vi "main_mg400_m1pro.vi"() -> ()   [LabVIEW 2017]
panel:
  out "error out 6":errorcluster
  in  "MoveL":bool
  out "error out 5":errorcluster
  out "error out 4":errorcluster
  out "error out 3":errorcluster
  out "Current SpeedFactor":dbl
  out "error out 2":errorcluster
  out "Error Log":string
  in  "GetErrorID":bool
  out "x value":string
  out "y value":string
  out "z value":string
  out "rx value":string
  out "j4 value":string
  out "j3 value":string
  out "j2 value":string
  out "j1 value":string
  in  "rx-":bool
  in  "z-":bool
  in  "y-":bool
  in  "x-":bool
  in  "rx+":bool
  in  "z+":bool
  in  "y+":bool
  in  "x+":bool
  in  "JointMovJ":bool
  in  "j4":dbl
  in  "j3":dbl
  in  "j2":dbl
  in  "j1":dbl
  in  "Reset Robot":bool
  in  "Feedback Port":string="30004"
  in  "Move Port":string="30003"
  in  "Dashboard Port":string="29999"
  in  "IP Address":string="192.168.5.1"
  in  "stop get state":bool
  out "state error out 2":errorcluster
  out "Robot mode":T1(ring)
  out "speed set string":string
  in  "j4-":bool
  in  "j3-":bool
  in  "j2-":bool
  in  "j1-":bool
  in  "j4+":bool
  in  "j3+":bool
  in  "j2+":bool
  in  "j1+":bool
  out "error out":errorcluster
  in  "stop connect":bool
  in  "Start trace":bool
  in  "tracePath":string
  in  "Stop move":bool
  in  "MoveJ":bool
  in  "rx":dbl
  in  "z":dbl
  in  "y":dbl
  in  "x":dbl
  in  "Speed confrim":bool
  in  "Speed Ratio":dbl=50.0
  in  "Emergency Stop":bool
  in  "Power up":bool
  out "Log":string
  in  "ClearError":bool
  in  "Enable Robot":bool
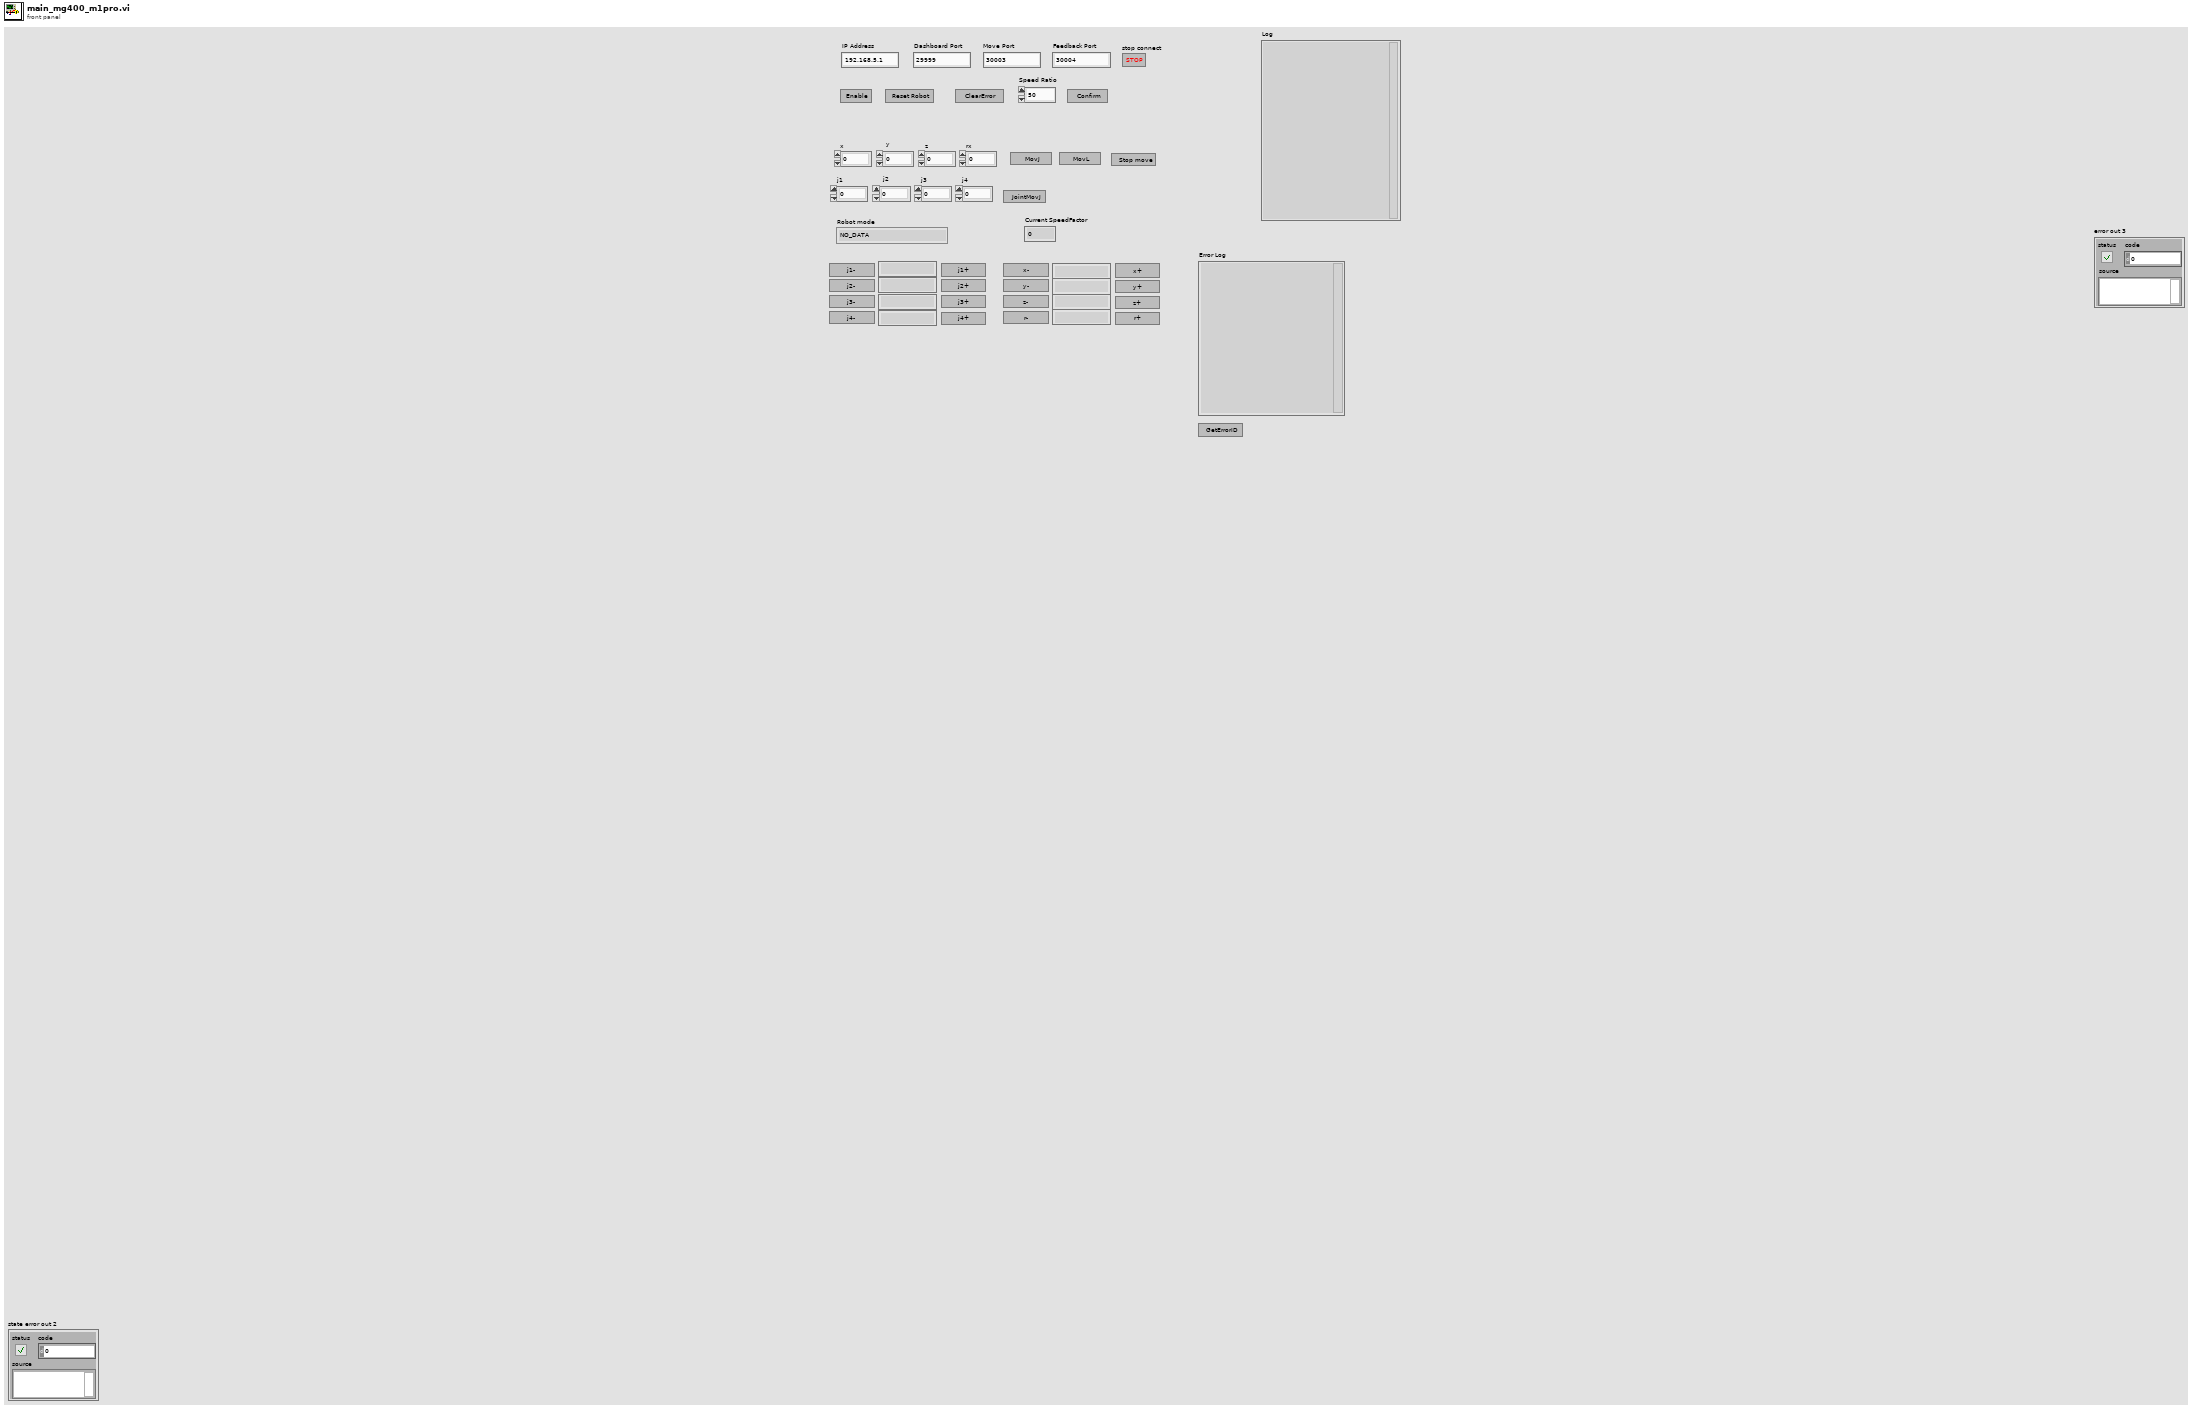
[diagram p1: front panel]
types:
  T1 = enum16{"NO_DATA", "ROBOT_MODE_INIT", "ROBOT_MODE_BRAKE_OPEN", "HOLD_BITS", "ROBOT_MODE_DISABLED", "ROBOT_MODE_ENABLE", "ROBOT_MODE_BACKDRIVE", "ROBOT_MODE_RUNNING", "ROBOT_MODE_RECORDING", "ROBOT_MODE_ERROR", "ROBOT_MODE_PAUSE", "ROBOT_MODE_JOG"}
  T2 = enum16{"Standard", "Buffered", "CRLF", "Immediate"}
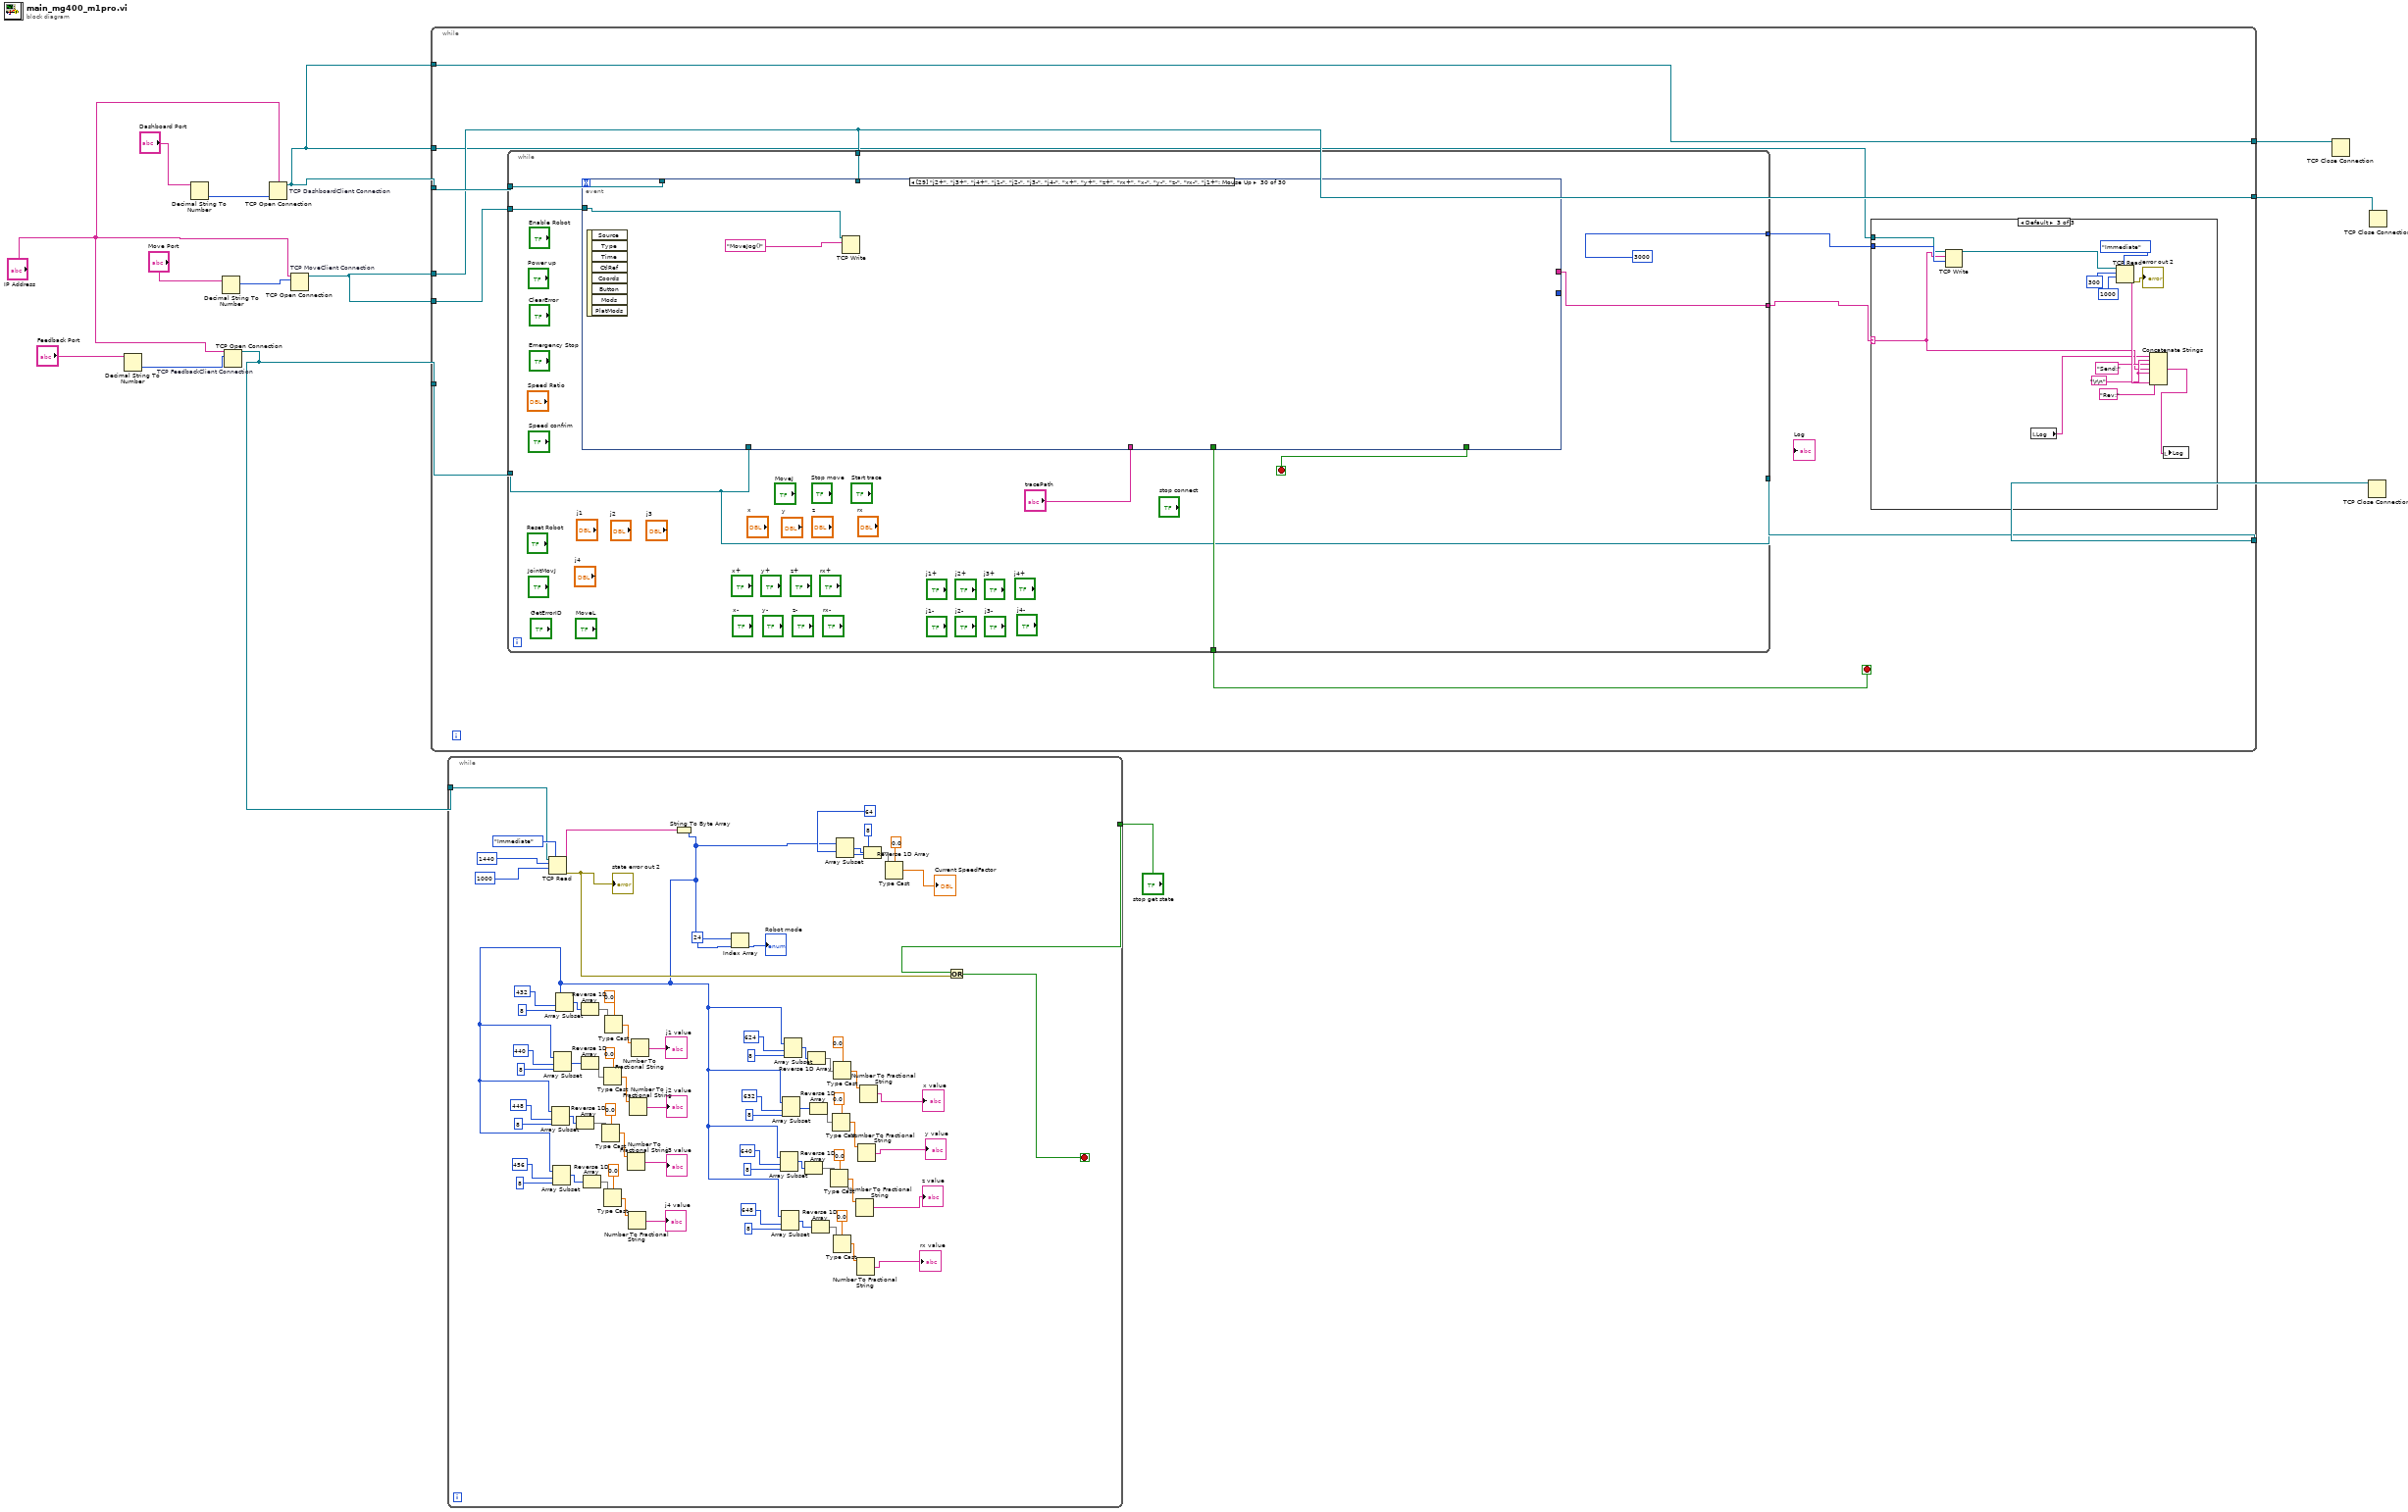
[diagram p0: block diagram]
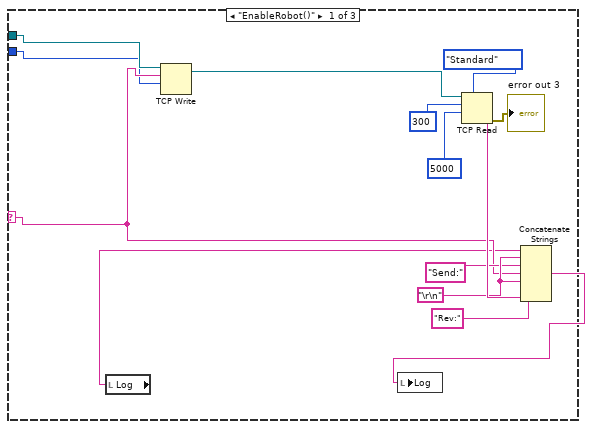
[diagram p2: hidden frame]
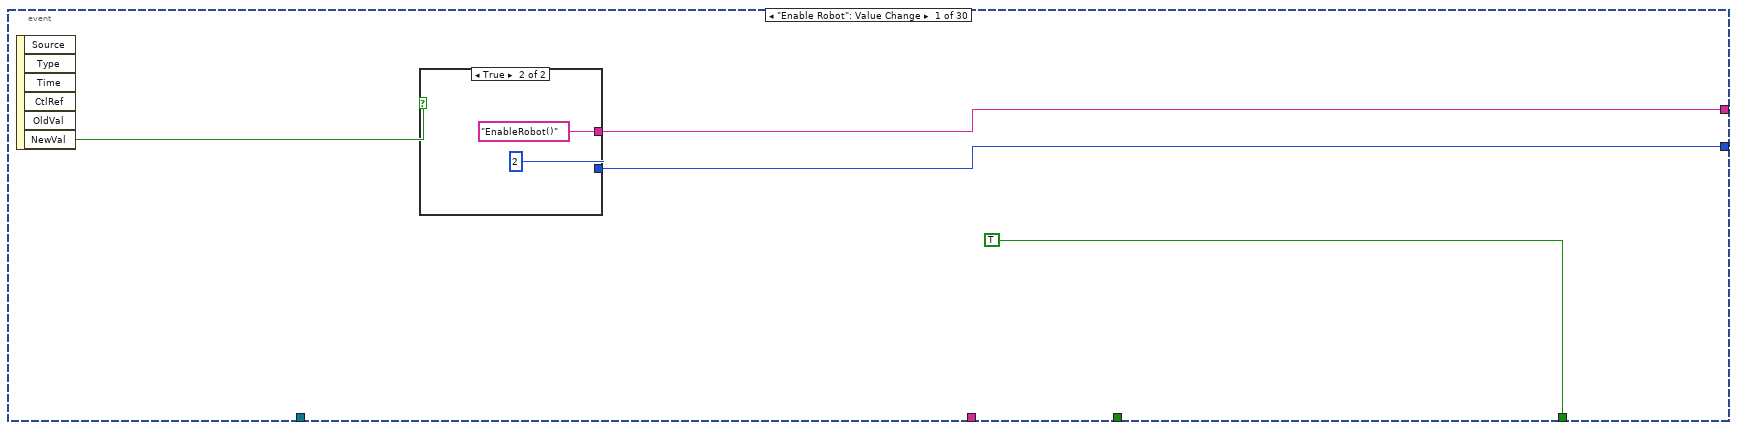
[diagram p4: hidden frame]
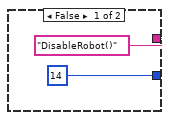
[diagram p5: hidden frame]
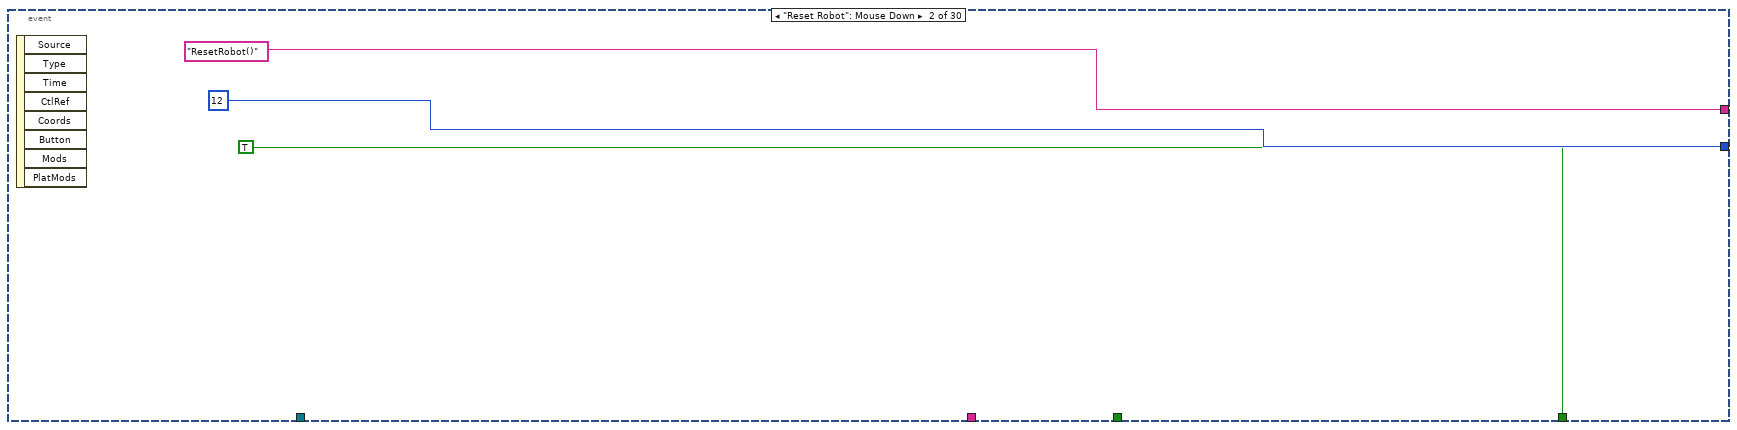
[diagram p6: hidden frame]
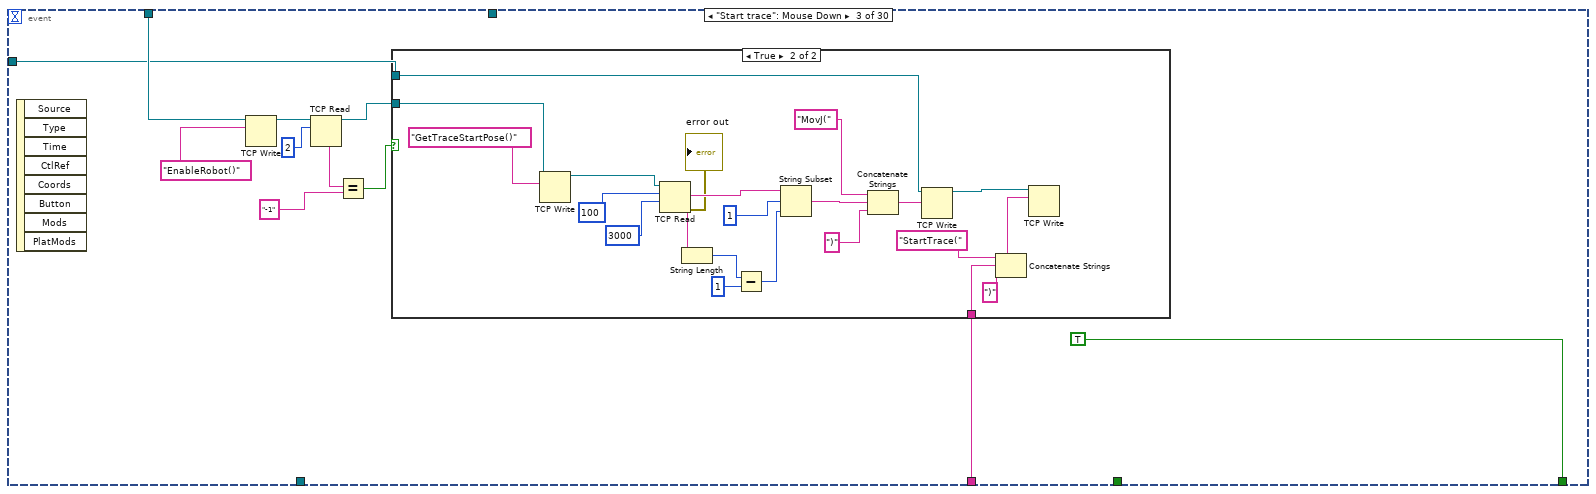
[diagram p7: hidden frame]
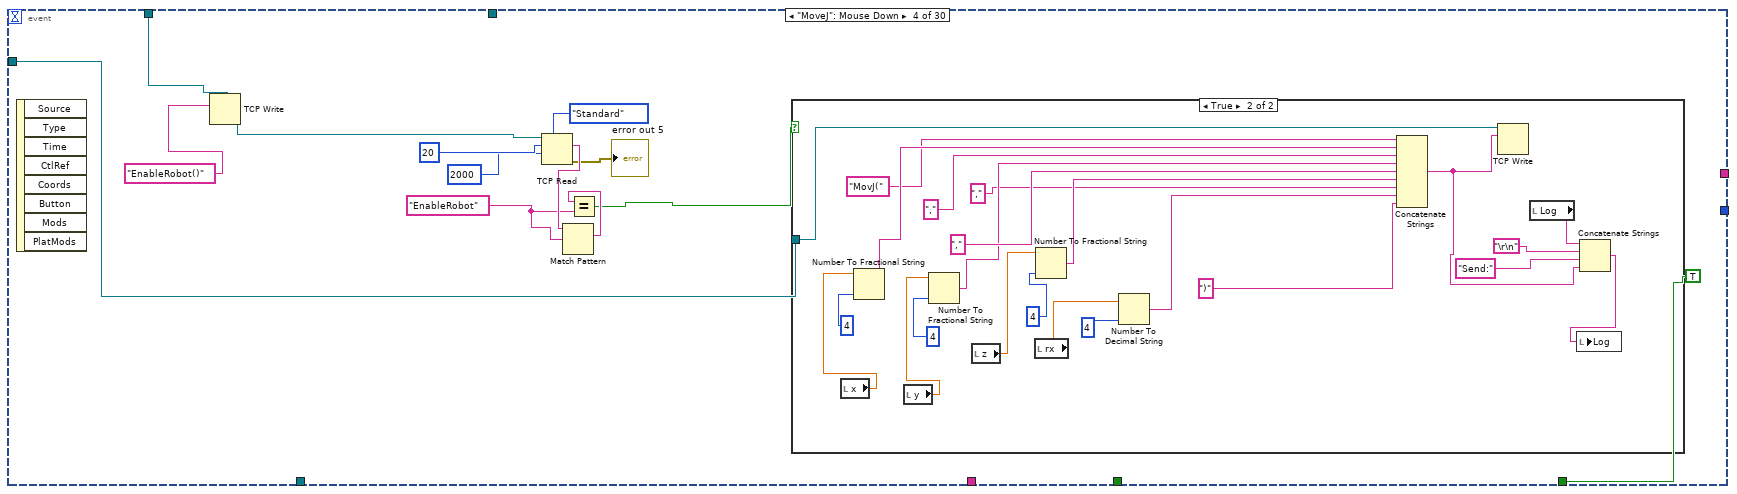
[diagram p9: hidden frame]
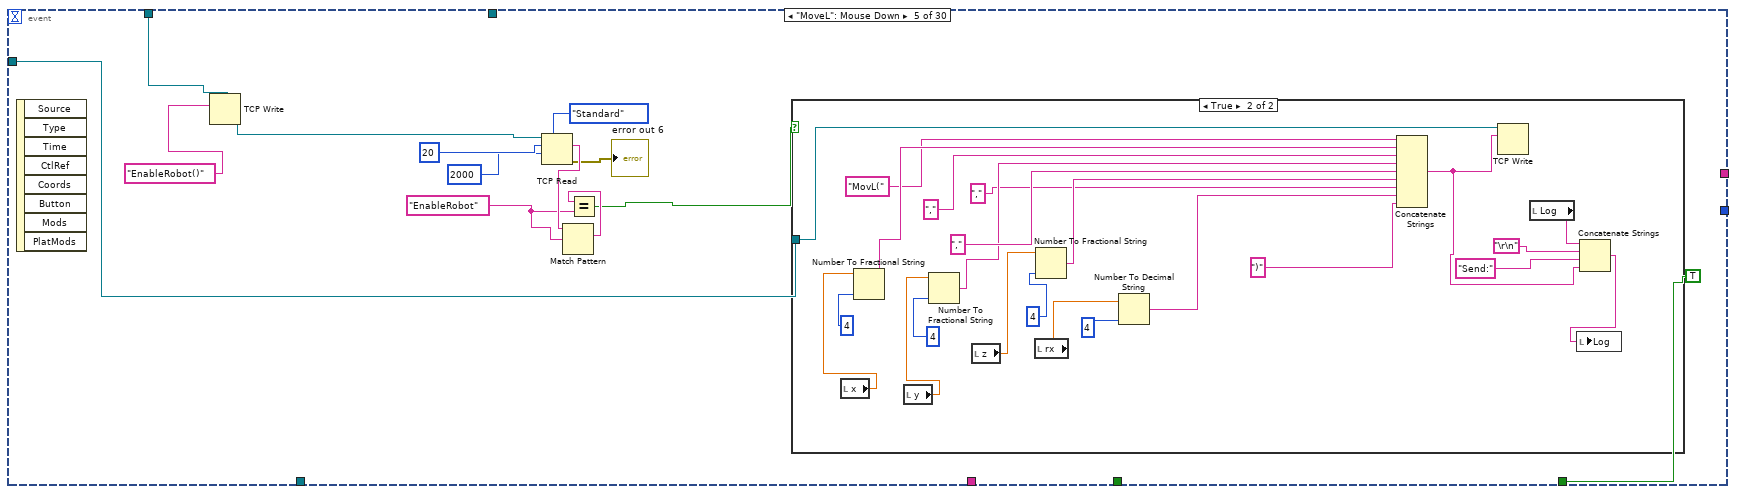
[diagram p11: hidden frame]
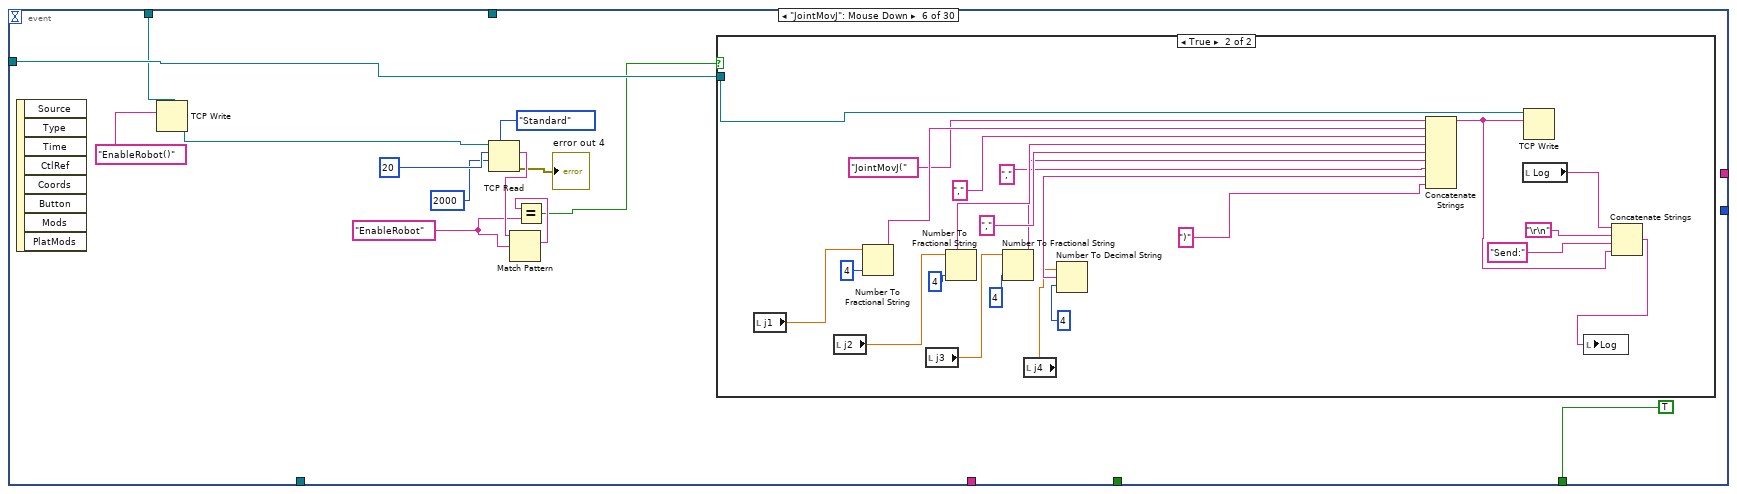
[diagram p13: hidden frame]
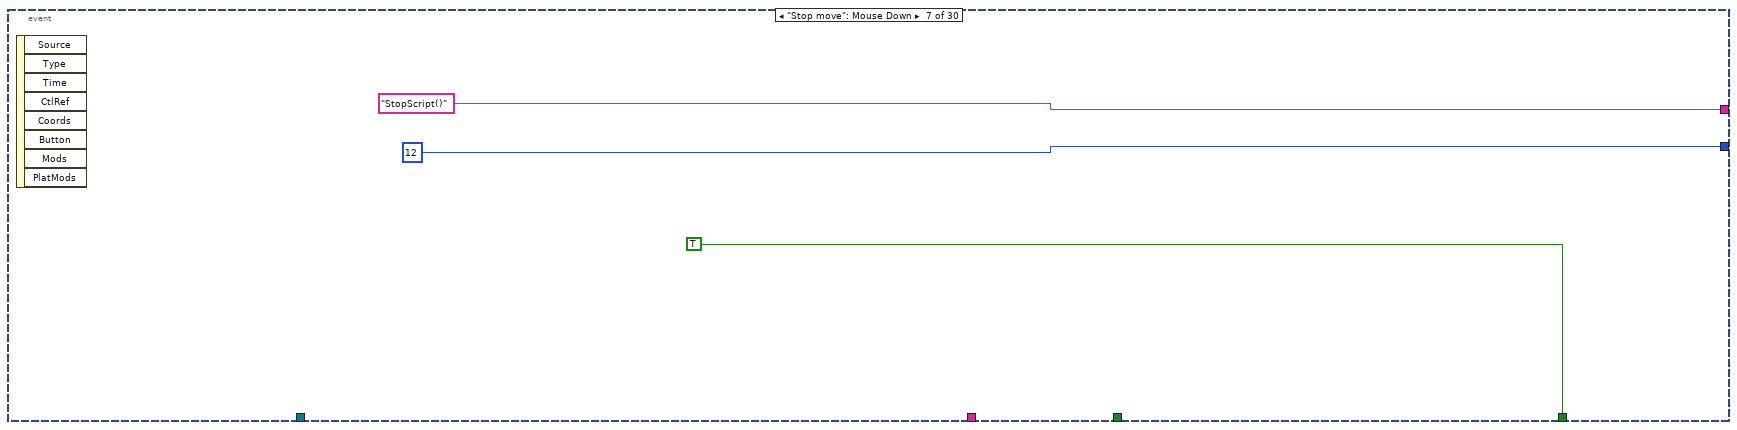
[diagram p15: hidden frame]
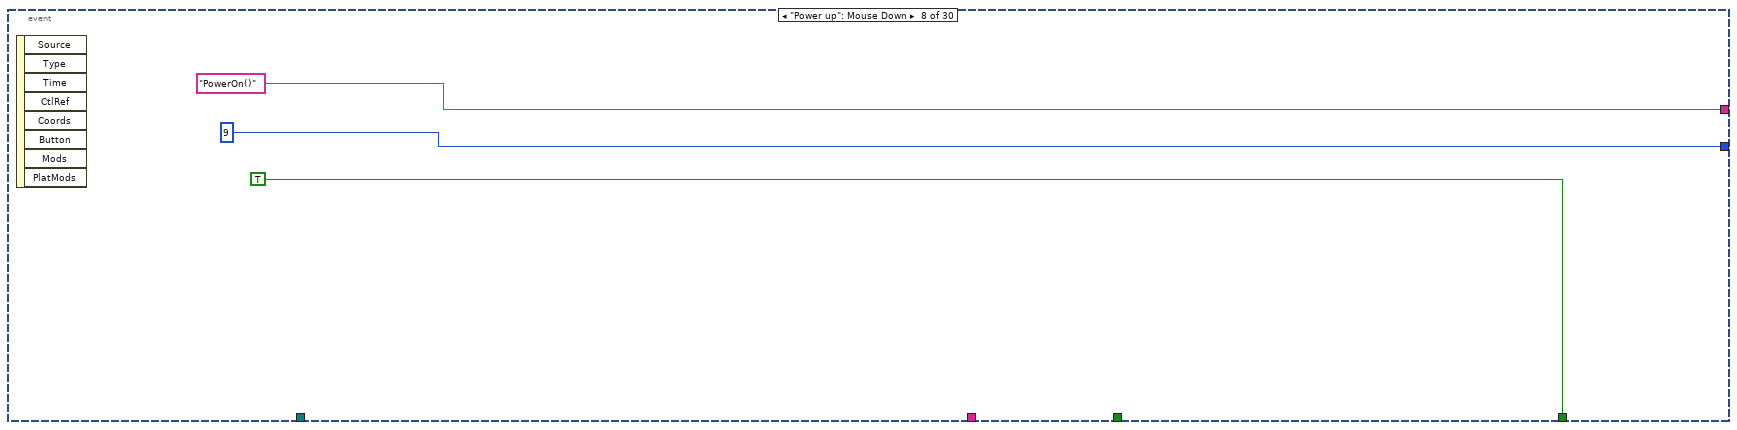
[diagram p16: hidden frame]
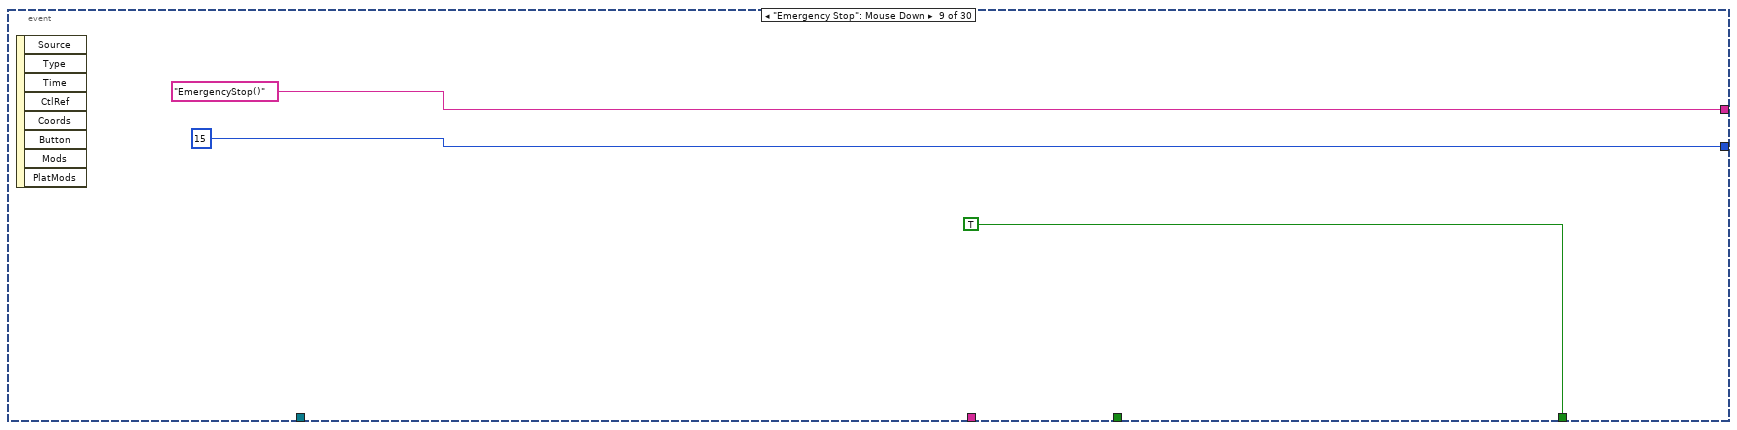
[diagram p17: hidden frame]
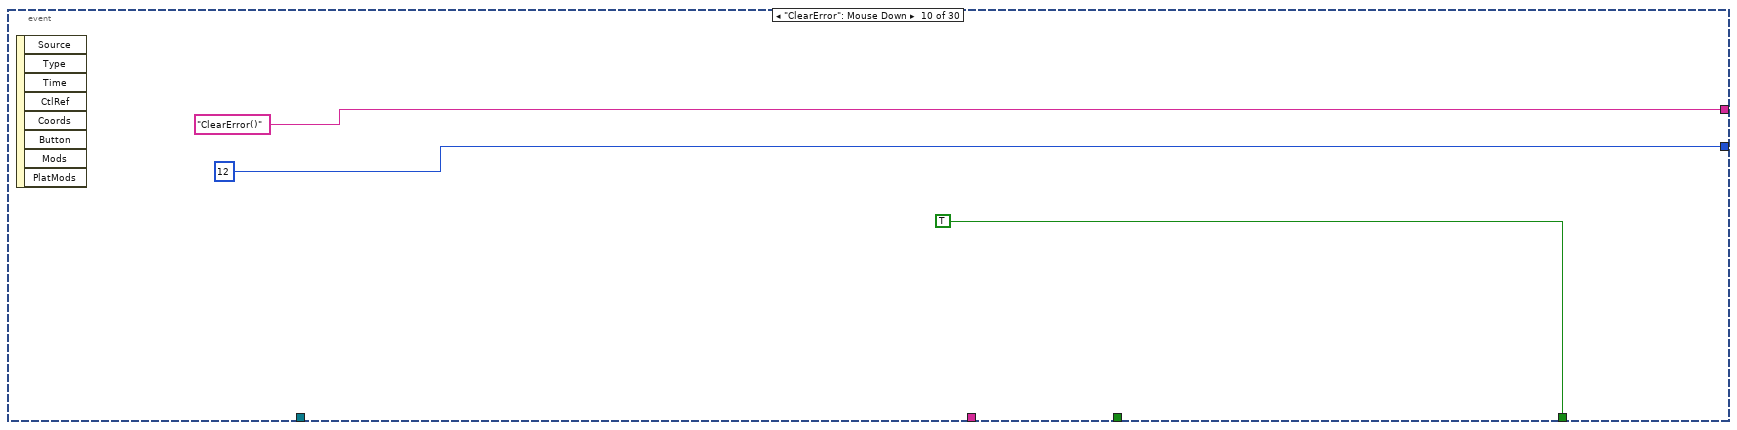
[diagram p18: hidden frame]
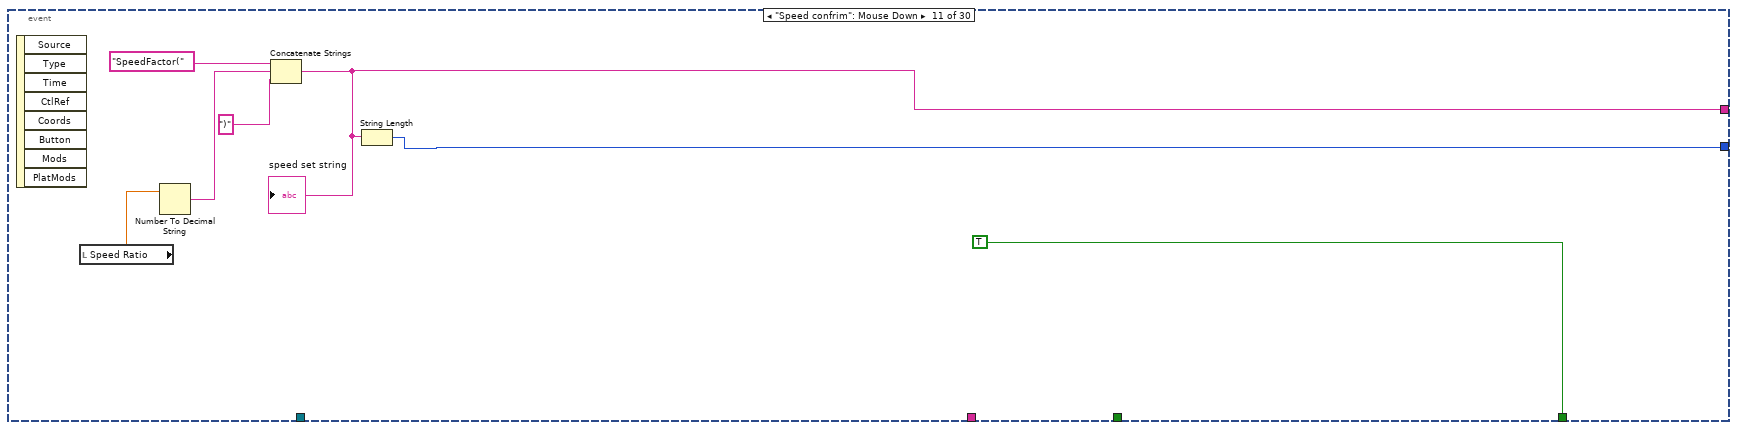
[diagram p19: hidden frame]
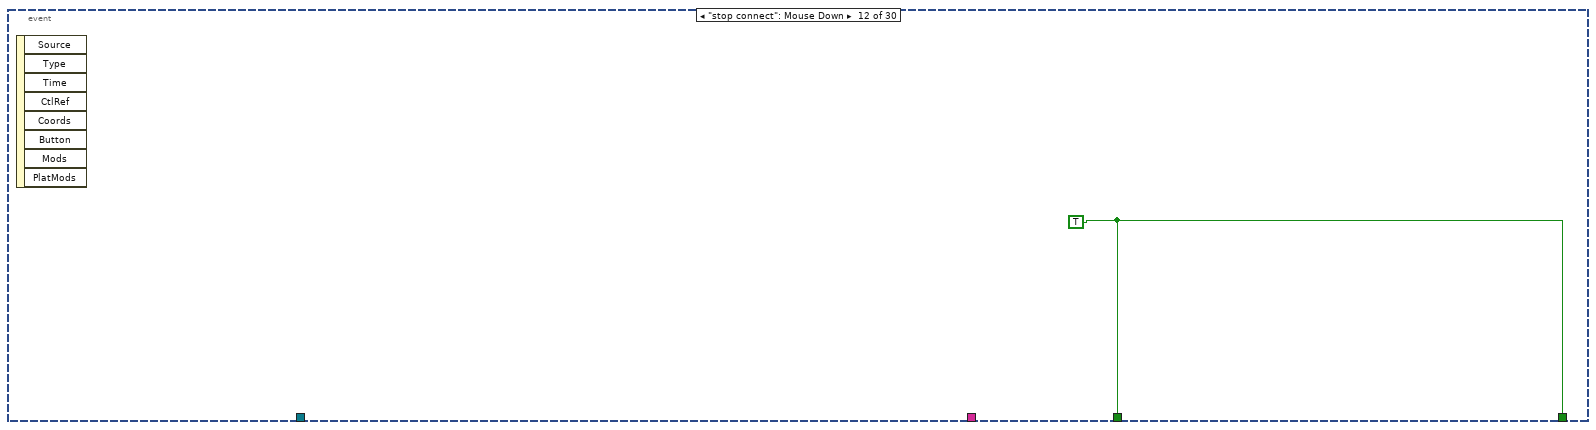
[diagram p20: hidden frame]
diagram:
  n1 = Decimal String To Number(string="Feedback Port") -> (number=w2:i32)  [unwired: 2 in, 1 out]
  n2 = Decimal String To Number(string="Dashboard Port") -> (number=w4:i32)  [unwired: 2 in, 1 out]
  n3 = Decimal String To Number(string="Move Port") -> (number=w3:i32)  [unwired: 2 in, 1 out]
  n4 = TCP Open Connection "TCP FeedbackClient Connection"(address="IP Address", remote port or service name=w2) -> (connection ID=w9:refnum<k5>)  [unwired: 3 in, 1 out]
  n5 = TCP Open Connection "TCP DashboardClient Connection"(address="IP Address", remote port or service name=w4) -> (connection ID=w1:refnum<k5>)  [unwired: 3 in, 1 out]
  n6 = TCP Open Connection "TCP MoveClient Connection"(address="IP Address", remote port or service name=w3) -> (connection ID=w12:refnum<k5>)  [unwired: 3 in, 1 out]
  n7 = while {
    tunnel: [w18] -> w14
    tunnel: w12 -> [w18]
    tunnel: [w24] -> w13
    tunnel: w1 -> [w24]
    tunnel: w1 -> [w23]
    tunnel: w12 -> [w22]
    tunnel: w9 -> [w20]
    tunnel: [w19] -> w11
    tunnel: w1 -> [w16]
    stop <- w21 stop-if-true
    n8 = while {
      tunnel: w23 -> [w61]
      tunnel: w22 -> [w60]
      tunnel: [w57] -> w21
      tunnel: w20 -> [w56]
      tunnel: [w56] -> w19
      tunnel: w18 -> [w55]
      tunnel: [w54] -> w15
      tunnel: [3000 ("timeout ms (25000)")] -> w17
      stop <- w58 stop-if-true
      n9 = event shown="[29] \"j2+\", \"j3+\", \"j4+\", \"j1-\", \"j2-\", \"j3-\", \"j4-\", \"x+\", \"y+\", \"z+\", \"rx+\", \"x-\", \"y-\", \"z-\", \"rx-\", \"j1+\": Mouse Up" {
        selector: _ -> [_ _ _ _ _ _ _ _ _ _ _ _ _ _ _ _ _ _ _ _ _ _ _ _ _ _ _ _ _ _]
        dyn-events: _ -> [_ _ _ _ _ _ _ _ _ _ _ _ _ _ _ _ _ _ _ _ _ _ _ _ _ _ _ _ _ _]
        timeout: _ -> [_ _ _ _ _ _ _ _ _ _ _ _ _ _ _ _ _ _ _ _ _ _ _ _ _ _ _ _ _ _]
        tunnel: [w62 "ResetRobot()" _ _ _ _ "StopScript()" "PowerOn()" "EmergencyStop()" "ClearError()" w226 _ _ _ _ _ _ _ _ _ _ _ _ _ _ _ _ _ _ _] -> w54
        tunnel: [w64 12 _ _ _ _ 12 9 15 12 w229 _ _ _ _ _ _ _ _ _ _ _ _ _ _ _ _ _ _ _] -> _
        tunnel: w61 -> [_ _ w78 w109 w145 w181 _ _ _ _ _ _ _ _ _ _ _ _ _ _ _ _ _ _ _ _ _ _ _ _]
        tunnel: w60 -> [_ _ w75 w117 w153 w188 _ _ _ _ _ _ _ w241 w243 w245 w247 w249 w251 w253 w255 w257 w259 w261 w263 w265 w267 w269 w271 w273]
        tunnel: "tracePath" -> [_ _ w74 _ _ _ _ _ _ _ _ _ _ _ _ _ _ _ _ _ _ _ _ _ _ _ _ _ _ _]
        tunnel: [TRUE TRUE TRUE TRUE TRUE TRUE TRUE TRUE TRUE TRUE TRUE w232 TRUE _ _ _ _ _ _ _ _ _ _ _ _ _ _ _ _ _] -> w58
        tunnel: [_ _ _ _ _ _ _ _ _ _ _ w232 _ _ _ _ _ _ _ _ _ _ _ _ _ _ _ _ _ _] -> w57
        tunnel: w56 -> [_ _ _ _ _ _ _ _ _ _ _ _ _ _ _ _ _ _ _ _ _ _ _ _ _ _ _ _ _ _]
        tunnel: w55 -> [_ _ _ _ _ _ _ _ _ _ _ _ w238 _ _ _ _ _ _ _ _ _ _ _ _ _ _ _ _ _]
        event "Enable Robot": Value Change {
          n10 = event-data() -> ("NewVal"=w65:bool)  [unwired: 1 in, 5 out]
          n11 = case shown="True" w65 {
            tunnel: ["DisableRobot()" "EnableRobot()"] -> w62
            tunnel: [14 2] -> w64
            frame False {
            }
            frame True {
            }
          }
        }
        event "Reset Robot": Mouse Down {
          n12 = event-data() -> ()  [unwired: 1 in, 8 out]
        }
        event "Start trace": Mouse Down {
          n13 = event-data() -> ()  [unwired: 1 in, 8 out]
          n14 = TCP Write(connection ID=w78, data in="EnableRobot()") -> (connection ID out=w83:refnum<k5>)  [unwired: 2 in, 2 out]
          n15 = TCP Read(connection ID=w83, bytes to read=2) -> (connection ID out=w76:refnum<k5>, data out=w80:string)  [unwired: 3 in, 1 out]
          n16 = Equal?(x=w80, y="-1") -> (x = y?=w77:bool)
          n17 = case shown="True" w77 {
            tunnel: w76 -> [_ w103]
            tunnel: w75 -> [_ w90]
            tunnel: w74 -> [_ w86]
            frame False {
            }
            frame True {
              n18 = TCP Write(connection ID=w103, data in="GetTraceStartPose()") -> (connection ID out=w101:refnum<k5>)  [unwired: 2 in, 2 out]
              n19 = TCP Read(connection ID=w101, bytes to read=100, 9:3000 ("timeout ms (25000)")) -> (data out=w98:string, error out=→"error out":errorcluster)  [unwired: 2 in, 1 out]
              n20 = String Length(string=w98) -> (length=w97:i32)
              n21 = Subtract(x=w97, y=1) -> (x-y=w95:i32)
              n22 = String Subset(string=w98, offset (0)=1, length (rest)=w95) -> (substring=w93:string)
              n23 = Concatenate Strings("MovJ(" ("string"), w93, ")" ("string")) -> (w91:string)
              n24 = TCP Write(connection ID=w90, data in=w91) -> (connection ID out=w89:refnum<k5>)  [unwired: 2 in, 2 out]
              n25 = Concatenate Strings("StartTrace(" ("string"), w86, ")" ("string")) -> (w87:string)
              n26 = TCP Write(connection ID=w89, data in=w87) -> ()  [unwired: 2 in, 3 out]
            }
          }
        }
        event "MoveJ": Mouse Down {
          w112 = "EnableRobot" ("y")
          n27 = event-data() -> ()  [unwired: 1 in, 8 out]
          n28 = TCP Write(connection ID=w109, data in="EnableRobot()") -> (connection ID out=w115:refnum<k5>)  [unwired: 2 in, 2 out]
          n29 = TCP Read(connection ID=w115, bytes to read=20, 7:T2."Standard" ("mode (standard)"), 9:2000 ("timeout ms (25000)")) -> (data out=w114:string, error out=→"error out 5":errorcluster)  [unwired: 1 in, 1 out]
          n30 = Match Pattern(string=w114, regular expression=w112) -> (match substring=w113:string)  [unwired: 1 in, 3 out]
          n31 = Equal?(x=w113, y=w112) -> (x = y?=w107:bool)
          n32 = case shown="True" w107 {
            tunnel: w117 -> [_ w140]
            frame False {
            }
            frame True {
              n33 = local read "x"() -> (w123:dbl)
              n34 = Number To Fractional String(number=w123, precision (6)=i16 4) -> (F-format string=w139:string)  [unwired: 2 in]
              n35 = local read "y"() -> (w124:dbl)
              n36 = Number To Fractional String(number=w124, precision (6)=i16 4) -> (F-format string=w135:string)  [unwired: 2 in]
              n37 = local read "z"() -> (w125:dbl)
              n38 = local read "rx"() -> (w126:dbl)
              n39 = Number To Fractional String(number=w125, precision (6)=i16 4) -> (F-format string=w129:string)  [unwired: 2 in]
              n40 = Number To Decimal String(number=w126, width (-)=i16 4 ("precision (6)")) -> (decimal integer string=w134:string)
              n41 = Concatenate Strings("MovJ(" ("string"), w139, "," ("string"), w135, "," ("string"), w129, "," ("string"), w134, ")" ("string")) -> (w119:string)
              n42 = TCP Write(connection ID=w140, data in=w119) -> ()  [unwired: 2 in, 3 out]
              n43 = local read "Log"() -> (w122:string)
              n44 = Concatenate Strings(w122, "\r\n", "Send:" ("string"), w119) -> (w118:string)
              n45 = local write "Log"(w118) -> ()
            }
          }
        }
        event "MoveL": Mouse Down {
          w148 = "EnableRobot" ("y")
          n46 = event-data() -> ()  [unwired: 1 in, 8 out]
          n47 = TCP Write(connection ID=w145, data in="EnableRobot()") -> (connection ID out=w151:refnum<k5>)  [unwired: 2 in, 2 out]
          n48 = TCP Read(connection ID=w151, bytes to read=20, 7:T2."Standard" ("mode (standard)"), 9:2000 ("timeout ms (25000)")) -> (data out=w150:string, error out=→"error out 6":errorcluster)  [unwired: 1 in, 1 out]
          n49 = Match Pattern(string=w150, regular expression=w148) -> (match substring=w149:string)  [unwired: 1 in, 3 out]
          n50 = Equal?(x=w149, y=w148) -> (x = y?=w143:bool)
          n51 = case shown="True" w143 {
            tunnel: w153 -> [_ w176]
            frame False {
            }
            frame True {
              n52 = local read "x"() -> (w159:dbl)
              n53 = Number To Fractional String(number=w159, precision (6)=i16 4) -> (F-format string=w175:string)  [unwired: 2 in]
              n54 = local read "y"() -> (w160:dbl)
              n55 = Number To Fractional String(number=w160, precision (6)=i16 4) -> (F-format string=w171:string)  [unwired: 2 in]
              n56 = local read "z"() -> (w161:dbl)
              n57 = local read "rx"() -> (w162:dbl)
              n58 = Number To Fractional String(number=w161, precision (6)=i16 4) -> (F-format string=w165:string)  [unwired: 2 in]
              n59 = Number To Decimal String(number=w162, width (-)=i16 4 ("precision (6)")) -> (decimal integer string=w170:string)
              n60 = Concatenate Strings("MovL(" ("string"), w175, "," ("string"), w171, "," ("string"), w165, "," ("string"), w170, ")" ("string")) -> (w155:string)
              n61 = TCP Write(connection ID=w176, data in=w155) -> ()  [unwired: 2 in, 3 out]
              n62 = local read "Log"() -> (w158:string)
              n63 = Concatenate Strings(w158, "\r\n", "Send:" ("string"), w155) -> (w154:string)
              n64 = local write "Log"(w154) -> ()
            }
          }
        }
        event "JointMovJ": Mouse Down {
          w183 = "EnableRobot" ("y")
          n65 = event-data() -> ()  [unwired: 1 in, 8 out]
          n66 = TCP Write(connection ID=w181, data in="EnableRobot()") -> (connection ID out=w187:refnum<k5>)  [unwired: 2 in, 2 out]
          n67 = TCP Read(connection ID=w187, bytes to read=20, 7:T2."Standard" ("mode (standard)"), 9:2000 ("timeout ms (25000)")) -> (data out=w185:string, error out=→"error out 4":errorcluster)  [unwired: 1 in, 1 out]
          n68 = Match Pattern(string=w185, regular expression=w183) -> (match substring=w184:string)  [unwired: 1 in, 3 out]
          n69 = Equal?(x=w184, y=w183) -> (x = y?=w182:bool)
          n70 = case shown="True" w182 {
            tunnel: w188 -> [_ w212]
            frame False {
            }
            frame True {
              n71 = local read "j1"() -> (w198:dbl)
              n72 = local read "j2"() -> (w196:dbl)
              n73 = Number To Fractional String(number=w198, precision (6)=i16 4) -> (F-format string=w211:string)  [unwired: 2 in]
              n74 = local read "j3"() -> (w197:dbl)
              n75 = Number To Fractional String(number=w196, precision (6)=i16 4) -> (F-format string=w207:string)  [unwired: 2 in]
              n76 = Number To Fractional String(number=w197, precision (6)=i16 4) -> (F-format string=w202:string)  [unwired: 2 in]
              n77 = local read "j4"() -> (w199:dbl)
              n78 = Number To Decimal String(number=w199, width (-)=i16 4 ("precision (6)")) -> (decimal integer string=w206:string)
              n79 = Concatenate Strings("JointMovJ(" ("string"), w211, "," ("string"), w207, "," ("string"), w202, "," ("string"), w206, ")" ("string")) -> (w193:string)
              n80 = local read "Log"() -> (w192:string)
              n81 = TCP Write(connection ID=w212, data in=w193) -> ()  [unwired: 2 in, 3 out]
              n82 = Concatenate Strings(w192, "\r\n", "Send:" ("string"), w193) -> (w191:string)
              n83 = local write "Log"(w191) -> ()
            }
          }
        }
        event "Stop move": Mouse Down {
          n84 = event-data() -> ()  [unwired: 1 in, 8 out]
        }
        event "Power up": Mouse Down {
          n85 = event-data() -> ()  [unwired: 1 in, 8 out]
        }
        event "Emergency Stop": Mouse Down {
          n86 = event-data() -> ()  [unwired: 1 in, 8 out]
        }
        event "ClearError": Mouse Down {
          n87 = event-data() -> ()  [unwired: 1 in, 8 out]
        }
        event "Speed confrim": Mouse Down {
          n88 = event-data() -> ()  [unwired: 1 in, 8 out]
          n89 = local read "Speed Ratio"() -> (w225:dbl)
          n90 = Number To Decimal String(number=w225) -> (decimal integer string=w231:string)  [unwired: 1 in]
          n91 = Concatenate Strings("SpeedFactor(", w231, ")") -> (w226:string)
          "speed set string" <- w226
          n92 = String Length(string=w226) -> (length=w229:i32)
        }
        event "stop connect": Mouse Down {
          w232 = TRUE
          n93 = event-data() -> ()  [unwired: 1 in, 8 out]
        }
        event "GetErrorID": Mouse Down {
          w236 = 3000 ("timeout ms (25000)")
          n94 = event-data() -> ()  [unwired: 1 in, 8 out]
          n95 = TCP Write(connection ID=w238, data in="GetErrorID()", 9:w236) -> (connection ID out=w237:refnum<k5>)  [unwired: 1 in, 2 out]
          n96 = TCP Read(connection ID=w237, bytes to read=128, 7:T2."Immediate" ("mode (standard)"), 9:w236) -> (data out=→"Error Log":string)  [unwired: 1 in, 2 out]
        }
        event "j1+": Mouse Down {
          n97 = event-data() -> ()  [unwired: 1 in, 8 out]
          n98 = TCP Write(connection ID=w241, data in="MoveJog(j1+)") -> ()  [unwired: 2 in, 3 out]
        }
        event "j2+": Mouse Down {
          n99 = event-data() -> ()  [unwired: 1 in, 8 out]
          n100 = TCP Write(connection ID=w243, data in="MoveJog(j2+)") -> ()  [unwired: 2 in, 3 out]
        }
        event "j3+": Mouse Down {
          n101 = event-data() -> ()  [unwired: 1 in, 8 out]
          n102 = TCP Write(connection ID=w245, data in="MoveJog(j3+)") -> ()  [unwired: 2 in, 3 out]
        }
        event "j4+": Mouse Down {
          n103 = event-data() -> ()  [unwired: 1 in, 8 out]
          n104 = TCP Write(connection ID=w247, data in="MoveJog(j4+)") -> ()  [unwired: 2 in, 3 out]
        }
        event "j1-": Mouse Down {
          n105 = event-data() -> ()  [unwired: 1 in, 8 out]
          n106 = TCP Write(connection ID=w249, data in="MoveJog(j1-)") -> ()  [unwired: 2 in, 3 out]
        }
        event "j2-": Mouse Down {
          n107 = event-data() -> ()  [unwired: 1 in, 8 out]
          n108 = TCP Write(connection ID=w251, data in="MoveJog(j2-)") -> ()  [unwired: 2 in, 3 out]
        }
        event "j3-": Mouse Down {
          n109 = event-data() -> ()  [unwired: 1 in, 8 out]
          n110 = TCP Write(connection ID=w253, data in="MoveJog(j3-)") -> ()  [unwired: 2 in, 3 out]
        }
        event "j4-": Mouse Down {
          n111 = event-data() -> ()  [unwired: 1 in, 8 out]
          n112 = TCP Write(connection ID=w255, data in="MoveJog(j4-)") -> ()  [unwired: 2 in, 3 out]
        }
        event "x+": Mouse Down {
          n113 = event-data() -> ()  [unwired: 1 in, 8 out]
          n114 = TCP Write(connection ID=w257, data in="MoveJog(x+)") -> ()  [unwired: 2 in, 3 out]
        }
        event "y+": Mouse Down {
          n115 = event-data() -> ()  [unwired: 1 in, 8 out]
          n116 = TCP Write(connection ID=w259, data in="MoveJog(y+)") -> ()  [unwired: 2 in, 3 out]
        }
        event "z+": Mouse Down {
          n117 = event-data() -> ()  [unwired: 1 in, 8 out]
          n118 = TCP Write(connection ID=w261, data in="MoveJog(z+)") -> ()  [unwired: 2 in, 3 out]
        }
        event "rx+": Mouse Down {
          n119 = event-data() -> ()  [unwired: 1 in, 8 out]
          n120 = TCP Write(connection ID=w263, data in="MoveJog(r+)") -> ()  [unwired: 2 in, 3 out]
        }
        event "x-": Mouse Down {
          n121 = event-data() -> ()  [unwired: 1 in, 8 out]
          n122 = TCP Write(connection ID=w265, data in="MoveJog(x-)") -> ()  [unwired: 2 in, 3 out]
        }
        event "y-": Mouse Down {
          n123 = event-data() -> ()  [unwired: 1 in, 8 out]
          n124 = TCP Write(connection ID=w267, data in="MoveJog(y-)") -> ()  [unwired: 2 in, 3 out]
        }
        event "z-": Mouse Down {
          n125 = event-data() -> ()  [unwired: 1 in, 8 out]
          n126 = TCP Write(connection ID=w269, data in="MoveJog(z-)") -> ()  [unwired: 2 in, 3 out]
        }
        event "rx-": Mouse Down {
          n127 = event-data() -> ()  [unwired: 1 in, 8 out]
          n128 = TCP Write(connection ID=w271, data in="MoveJog(r-)") -> ()  [unwired: 2 in, 3 out]
        }
        event "j2+", "j3+", "j4+", "j1-", "j2-", "j3-", "j4-", "x+", "y+", "z+", "rx+", "x-", "y-", "z-", "rx-", "j1+": Mouse Up {
          n129 = event-data() -> ()  [unwired: 1 in, 8 out]
          n130 = TCP Write(connection ID=w273, data in="MoveJog()") -> ()  [unwired: 2 in, 3 out]
        }
      }
    }
    n131 = case shown="Default" w15 {
      tunnel: w17 -> [w27 _ w43]
      tunnel: w16 -> [w28 _ w42]
      selector: w15 -> [w29 _ w41]
      frame "EnableRobot()" {
        w35 = "\r\n"
        n132 = local read "Log"() -> (w26:string)
        n133 = TCP Write(connection ID=w28, data in=w29, 9:w27) -> (connection ID out=w36:refnum<k5>)  [unwired: 1 in, 2 out]
        n134 = TCP Read(connection ID=w36, bytes to read=300, 7:T2."Standard" ("mode (standard)"), 9:5000 ("timeout ms (25000)")) -> (data out=w37:string, error out=→"error out 3":errorcluster)  [unwired: 1 in, 1 out]
        n135 = Concatenate Strings(w26, w35, "Send:" ("string"), w29, w35, "Rev:" ("string"), w37) -> (w25:string)
        n136 = local write "Log"(w25) -> ()
      }
      frame "" {
      }
      frame Default {
        w49 = "\r\n"
        n137 = TCP Write(connection ID=w42, data in=w41, 9:w43) -> (connection ID out=w50:refnum<k5>)  [unwired: 1 in, 2 out]
        n138 = local read "Log"() -> (w39:string)
        n139 = TCP Read(connection ID=w50, bytes to read=300, 7:T2."Immediate" ("mode (standard)"), 9:1000 ("timeout ms (25000)")) -> (data out=w51:string, error out=→"error out 2":errorcluster)  [unwired: 1 in, 1 out]
        n140 = Concatenate Strings(w39, w49, "Send:" ("string"), w41, w49, "Rev:" ("string"), w51) -> (w40:string)
        n141 = local write "Log"(w40) -> ()
      }
    }
  }
  n142 = while {
    tunnel: w9 -> [w344]
    tunnel: "stop get state" -> [w341]
    stop <- w340 stop-if-true
    n143 = TCP Read(connection ID=w344, bytes to read=1440, 7:T2."Immediate" ("mode (standard)"), 9:1000 ("timeout ms (25000)")) -> (data out=w342:string, error out=w339:errorcluster)  [unwired: 1 in, 1 out]
    "state error out 2" <- w339
    n144 = String To Byte Array(string=w342) -> (unsigned byte array=w275:u8[])
    n145 = Array Subset(array=w275, index=448, length=8) -> (w314:u8[])
    n146 = Array Subset(array=w275, index=456, length=8) -> (w312:u8[])
    n147 = Array Subset(array=w275, index=440, length=8) -> (w315:u8[])
    n148 = Array Subset(array=w275, index=432, length=8) -> (w318:u8[])
    n149 = Reverse 1D Array(array=w314) -> (reversed array=w313:u8[])
    n150 = Reverse 1D Array(array=w318) -> (reversed array=w317:u8[])
    n151 = Reverse 1D Array(array=w315) -> (reversed array=w316:u8[])
    n152 = Reverse 1D Array(array=w312) -> (reversed array=w311:u8[])
    n153 = Type Cast(type=0.0, x=w313) -> (*(type *) &x=w325:dbl)
    n154 = Type Cast(type=0.0, x=w316) -> (*(type *) &x=w330:dbl)
    n155 = Type Cast(type=0.0, x=w311) -> (*(type *) &x=w321:dbl)
    n156 = Type Cast(type=0.0, x=w317) -> (*(type *) &x=w335:dbl)
    n157 = Number To Fractional String(number=w325) -> (F-format string=→"j3 value":string)  [unwired: 3 in]
    n158 = Number To Fractional String(number=w321) -> (F-format string=→"j4 value":string)  [unwired: 3 in]
    n159 = Number To Fractional String(number=w330) -> (F-format string=→"j2 value":string)  [unwired: 3 in]
    n160 = Number To Fractional String(number=w335) -> (F-format string=→"j1 value":string)  [unwired: 3 in]
    n161 = Index Array(array=w275, index=24) -> (element=→"Robot mode":u8)
    n162 = Array Subset(array=w275, index=640, length=8) -> (w292:u8[])
    n163 = Array Subset(array=w275, index=648, length=8) -> (w290:u8[])
    n164 = Array Subset(array=w275, index=632, length=8) -> (w293:u8[])
    n165 = Array Subset(array=w275, index=624, length=8) -> (w284:u8[])
    n166 = Reverse 1D Array(array=w292) -> (reversed array=w291:u8[])
    n167 = Reverse 1D Array(array=w284) -> (reversed array=w283:u8[])
    n168 = Reverse 1D Array(array=w293) -> (reversed array=w294:u8[])
    n169 = Reverse 1D Array(array=w290) -> (reversed array=w289:u8[])
    n170 = Type Cast(type=0.0, x=w291) -> (*(type *) &x=w299:dbl)
    n171 = Type Cast(type=0.0, x=w294) -> (*(type *) &x=w303:dbl)
    n172 = Type Cast(type=0.0, x=w289) -> (*(type *) &x=w295:dbl)
    n173 = Type Cast(type=0.0, x=w283) -> (*(type *) &x=w307:dbl)
    n174 = Array Subset(array=w275, index=64, length=8) -> (w278:u8[])
    n175 = Number To Fractional String(number=w299) -> (F-format string=→"z value":string)  [unwired: 3 in]
    n176 = Number To Fractional String(number=w295) -> (F-format string=→"rx value":string)  [unwired: 3 in]
    n177 = Number To Fractional String(number=w303) -> (F-format string=→"y value":string)  [unwired: 3 in]
    n178 = Number To Fractional String(number=w307) -> (F-format string=→"x value":string)  [unwired: 3 in]
    n179 = Reverse 1D Array(array=w278) -> (reversed array=w277:u8[])
    n180 = Type Cast(type=0.0, x=w277) -> (*(type *) &x=→"Current SpeedFactor":dbl)
    n181 = Or(x=w341, y=w339) -> (x .or. y?=w340:bool)
  }
  n182 = TCP Close Connection(connection ID=w13) -> ()  [unwired: 2 in, 2 out]
  n183 = TCP Close Connection(connection ID=w11) -> ()  [unwired: 2 in, 2 out]
  n184 = TCP Close Connection(connection ID=w14) -> ()  [unwired: 2 in, 2 out]
